vi "Periodic Tasks.vi"(8 "error in":errorcluster) -> ()   [LabVIEW 2019]
doc: "This VI runs in parallel to other tasks. It can contain as many user-defined periodic loops as you need. These can carry out PID or other sorts of timed response."
uses:
  <vilib>/Rock Robotics/WPI/DriverStation/WPI_DriverStationRobotMode2.ctl
  <vilib>/Rock Robotics/WPI/Utilities/WPI_GetSetVariantRefNum.vi
  Robot Global Data.vi
  <vilib>/Rock Robotics/Network Tables/NT Write Numeric Array.vi
  <vilib>/Rock Robotics/WPI/RobotDrive/WPI_RobotDriveArcadeDrive_Standard(NoSaturation).vi
  <vilib>/Rock Robotics/Network Tables/NT Write String.vi
  <vilib>/Rock Robotics/Network Tables/NT Write Number.vi
panel:
  in  "Yellow":cluster{"R":dbl, "G":dbl, "B":dbl}
  in  "Blue":cluster{"R":dbl, "G":dbl, "B":dbl}
  in  "Green":cluster{"R":dbl, "G":dbl, "B":dbl}
  in  "Red":cluster{"R":dbl, "G":dbl, "B":dbl}
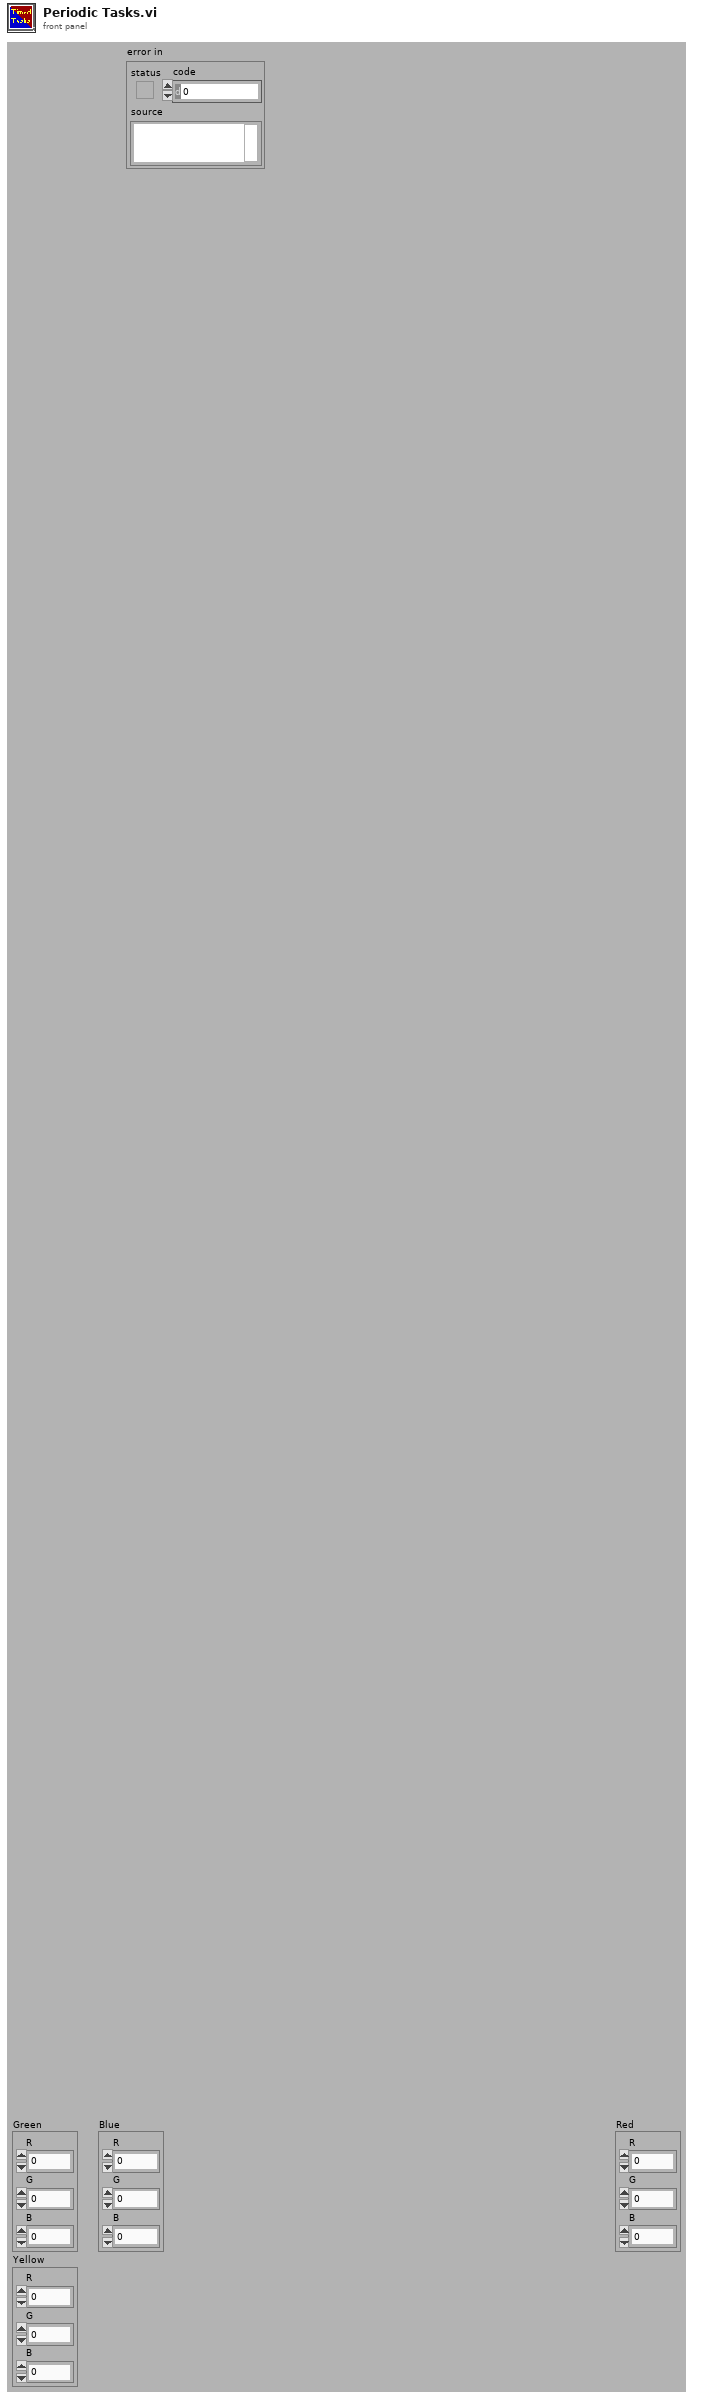
[diagram p1: front panel]
types:
  T1 = typedef "WPI_RobotDriveDevRef.ctl" = cluster{"DevStatus":errorcluster, "Motors[]":T2[], "Square Inputs":bool, "Max Output":dbl}
  T2 = typedef "WPI_MotorControlDeviceRef.ctl" = cluster{"DeviceStatus":errorcluster, "Type":T3, "PWM":cluster{"PWM Channel":T4, "DeadBand":T5}, "CAN":cluster{"Device Number":u8, "SetOutput VI Ref":variant, "GetOutput VI Ref":variant, "Enable VI Ref":variant, "Disable VI Ref":variant, "Data":variant}, "Invert":bool, "DIO PWM":cluster{"PWM \"Enable\" Channel":T4, "DIOChannel":T6, "PWM Rate":dbl}}
  T3 = typedef "WPI_MotorControlType.ctl" = enum16{"PWM", "CAN", "DIO PWM"}
  T4 = typedef "FPGA_DIOPWMChannel.ctl" = enum8{"PWM 0", "PWM 1", "PWM 2", "PWM 3", "PWM 4", "PWM 5", "PWM 6", "PWM 7", "PWM 8", "PWM 9", "PWM MXP 0", "PWM MXP 1", "PWM MXP 2", "PWM MXP 3", "PWM MXP 4", "PWM MXP 5", "PWM MXP 6", "PWM MXP 7", "PWM MXP 8", "PWM MXP 9", "Invalid"}
  T5 = typedef "WPI_PWMDeadband.ctl" = cluster{"Name":string, "maxPositivePwm":i32, "minPositivePwm":i32, "centerPwm":i32, "maxNegativePwm":i32, "minNegativePwm":i32, "angularRange":u16}
  T6 = typedef "FPGA_DIOChannel.ctl" = enum8{"DIO 0", "DIO 1", "DIO 2", "DIO 3", "DIO 4", "DIO 5", "DIO 6", "DIO 7", "DIO 8", "DIO 9", "DIO MXP 0", "DIO MXP 1", "DIO MXP 2", "DIO MXP 3", "DIO MXP 4", "DIO MXP 5", "DIO MXP 6", "DIO MXP 7", "DIO MXP 8", "DIO MXP 9", "DIO MXP 10", "DIO MXP 11", "DIO MXP 12", "DIO MXP 13", "DIO MXP 14", "DIO MXP 15", "SPI Port CS1", "SPI Port CS2", "SPI Port CS3", "SPI Port MISO", "SPI Port MOSI", "Invalid"}
  T7 = typedef "WPI_JoystickDevRef.ctl" = cluster{"Device":T8}
  T8 = typedef "WPI_JoystickDeviceEnum.ctl" = enum16{"USB 0", "USB 1", "USB 2", "USB 3", "USB 4", "USB 5"}
  T9 = cluster{"JoystickDevRef":T7, "RobotDriveDevRef":T1}
  T10 = typedef "Color Sensor V3 DevRef.ctl" = cluster{"I2CDevRef":T11}
  T11 = typedef "WPI_I2CDevRef.ctl" = cluster{"DevStatus":errorcluster, "Device Address":u8, "Handle":i32, "I2C Bus":T12}
  T12 = typedef "i2c_bus.ctl" = enum16{"I2C On-Board", "I2C MXP", "Invalid"}
  T13 = typedef "WPI_DriverStationRobotMode2.ctl" = enum16{"Autonomous Disabled", "Autonomous Enabled", "Teleop Disabled", "Teleop Enabled", "Disconnected", "Finish", "Test Disabled", "Test Enabled", "Emergency Stopped"}
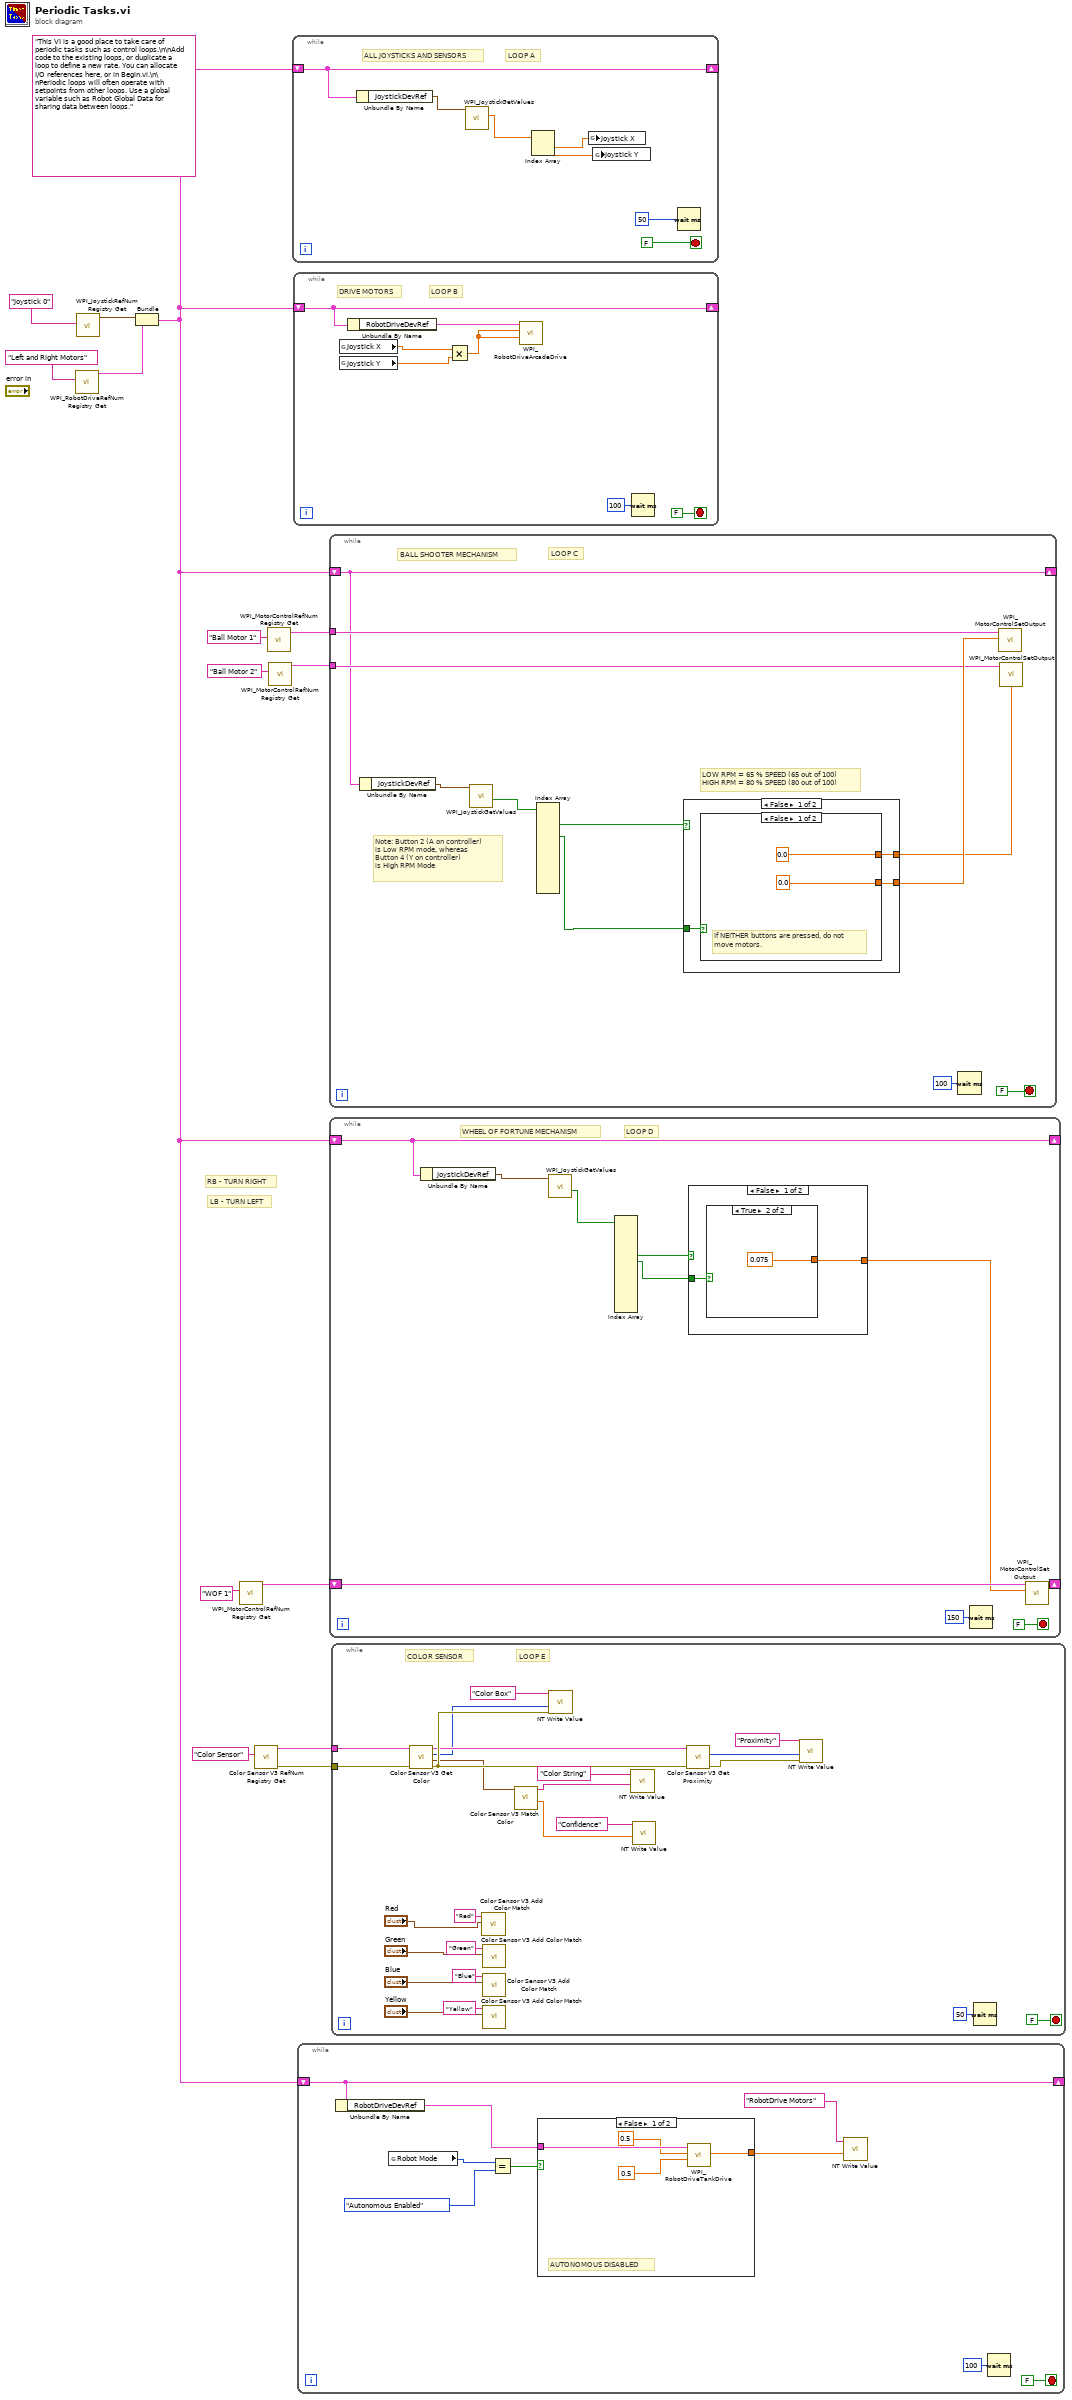
[diagram p0: block diagram]
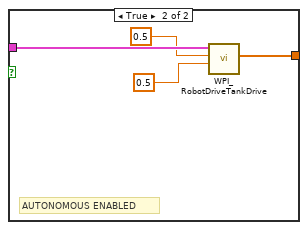
[diagram p2: hidden frame]
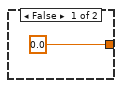
[diagram p3: hidden frame]
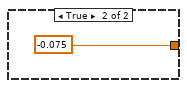
[diagram p4: hidden frame]
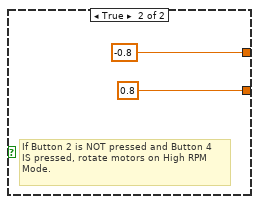
[diagram p5: hidden frame]
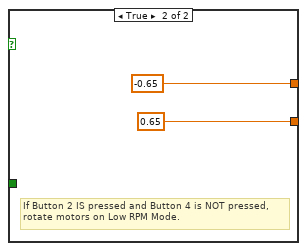
[diagram p6: hidden frame]
diagram:
  (unwired) "This VI is a good place to take care of periodic tasks such as control loops.\n\nAdd code to the existing loops, or duplicate a loop to define a new rate. You can allocate I/O references here, or in Begin.vi.\n\nPeriodic loops will often operate with setpoints from other loops. Use a global variable such as Robot Global Data for sharing data between loops."
  # "LB - TURN LEFT"
  # "RB - TURN RIGHT"
  n1 = call <vilib>:"WPI_RobotDriveRefNum Registry Get.vi"("refnum name"="Left and Right Motors") -> ("RobotDriveDevRef"=w11:T1)  [unwired: 1 in, 9 out]
  n2 = call <vilib>:"WPI_JoystickRefNum Registry Get.vi"("refnum name"="Joystick 0") -> ("JoystickDevRef"=w12:T7)  [unwired: 1 in, 9 out]
  n3 = Bundle("JoystickDevRef"=w12, "RobotDriveDevRef"=w11) -> (w1:T9)  [unwired: 1 out]
  n4 = call <vilib>:"WPI_MotorControlRefNum Registry Get.vi"("refnum name"="WOF 1") -> ("MotorControlDevRef"=w5:T2)  [unwired: 9 in, 1 out]
  n5 = call <vilib>:"Color Sensor V3 RefNum Registry Get.vi"("refnum name"="Color Sensor") -> ("error out"=w2:errorcluster, "ColorSensorDevRef"=w4:T10)  [unwired: 9 in]
  n6 = call <vilib>:"WPI_MotorControlRefNum Registry Get.vi"("refnum name"="Ball Motor 1") -> ("MotorControlDevRef"=w8:T2)  [unwired: 9 in, 1 out]
  n7 = call <vilib>:"WPI_MotorControlRefNum Registry Get.vi"("refnum name"="Ball Motor 2") -> ("MotorControlDevRef"=w7:T2)  [unwired: 9 in, 1 out]
  n8 = while {
    shift-right: [w20] -> _
    shift-left: w1 -> [w20]
    stop <- FALSE stop-if-true
    # "LOOP A"
    # "ALL JOYSTICKS AND SENSORS"
    n9 = Unbundle By Name(w20) -> ("JoystickDevRef"=w19:T7)
    n10 = call <vilib>:"WPI_JoystickGetValues.vi"("JoystickDevRef"=w19) -> ("Axes"=w18:dbl[])  [unwired: 6 in, 4 out]
    n11 = Index Array(array=w18) -> (element #1=w16:dbl, element #2=w17:dbl)  [unwired: 2 in]
    n12 = global write "Robot Global Data.vi" "Joystick X"(w16) -> ()
    n13 = global write "Robot Global Data.vi" "Joystick Y"(w17) -> ()
    n14 = Wait (ms)(milliseconds to wait=u32 50) -> ()  [unwired: 1 out]
  }
  n15 = while {
    shift-right: [w26] -> _
    shift-left: w1 -> [w26]
    stop <- FALSE stop-if-true
    # "LOOP B"
    # "DRIVE MOTORS"
    n16 = global read "Robot Global Data.vi" "Joystick X"() -> (w22:dbl)
    n17 = global read "Robot Global Data.vi" "Joystick Y"() -> (w23:dbl)
    n18 = Unbundle By Name(w26) -> ("RobotDriveDevRef"=w25:T1)
    n19 = Multiply(x=w22, y=w23) -> (x*y=w24:dbl)
    n20 = call-poly <vilib>:"WPI_RobotDriveArcadeDrive.vi"("Y axis value"=w24, "X axis value"=w24, "RobotDriveDevRef"=w25) -> ()  [unwired: 6 in, 3 out]
    n21 = Wait (ms)(milliseconds to wait=u32 100) -> ()  [unwired: 1 out]
  }
  n22 = while {
    shift-right: [w37] -> _
    shift-left: w1 -> [w37]
    stop <- FALSE stop-if-true
    n23 = Unbundle By Name(w37) -> ("RobotDriveDevRef"=w33:T1)
    n24 = global read "Robot Global Data.vi" "Robot Mode"() -> (w36:T13)
    n25 = Equal?(x=w36, y=WPI_DriverStationRobotMode2."Autonomous Enabled") -> (x = y?=w35:bool)
    n26 = case shown="False" w35 {
      tunnel: w33 -> [w40 w44]
      tunnel: [w41 w45] -> w29
      frame False {
        # "AUTONOMOUS DISABLED"
        n27 = call <vilib>:"WPI_RobotDriveTankDrive.vi"("Right axis value"=0.5, "Left axis value"=0.5, "RobotDriveDevRef"=w40) -> ("Motor Values"=w41:dbl[])  [unwired: 6 in, 2 out]
      }
      frame True {
        # "AUTONOMOUS ENABLED"
        n28 = call <vilib>:"WPI_RobotDriveTankDrive.vi"("Right axis value"=0.5, "Left axis value"=0.5, "RobotDriveDevRef"=w44) -> ("Motor Values"=w45:dbl[])  [unwired: 6 in, 2 out]
      }
    }
    n29 = call-poly <vilib>:"NT Write Value.vi"("Numeric Array"=w29, "Name"="RobotDrive Motors") -> ()  [unwired: 9 in, 1 out]
    n30 = Wait (ms)(milliseconds to wait=u32 100) -> ()  [unwired: 1 out]
  }
  n31 = while {
    shift-right: [w50] -> _
    shift-left: w1 -> [w50]
    tunnel: w8 -> [w54]
    tunnel: w7 -> [w51]
    stop <- FALSE stop-if-true
    # "LOW RPM = 65 % SPEED (65 out of 100)\nHIGH RPM = 80 % SPEED (80 out of 100)"
    # "LOOP C"
    # "Note: Button 2 (A on controller) \nis Low RPM mode, whereas \nButton 4 (Y on controller)\nis High RPM Mode"
    # "BALL SHOOTER MECHANISM"
    n32 = Unbundle By Name(w50) -> ("JoystickDevRef"=w49:T7)
    n33 = call <vilib>:"WPI_JoystickGetValues.vi"("JoystickDevRef"=w49) -> ("Buttons"=w48:bool[])  [unwired: 6 in, 4 out]
    n34 = Index Array(array=w48) -> (element #2=w46:bool, element #4=w47:bool)  [unwired: 13 in, 11 out]
    n35 = case shown="False" w46 {
      tunnel: [w59 0.65 ("Output")] -> w53
      tunnel: [w58 -0.65 ("Output")] -> w52
      tunnel: w47 -> [w57 _]
      frame False {
        n36 = case shown="False" w57 {
          tunnel: [0.0 ("Output") 0.8 ("Output")] -> w59
          tunnel: [0.0 ("Output") -0.8 ("Output")] -> w58
          frame False {
            # "If NEITHER buttons are pressed, do not\nmove motors."
          }
          frame True {
            # "If Button 2 is NOT pressed and Button 4\nIS pressed, rotate motors on High RPM\nMode."
          }
        }
      }
      frame True {
        # "If Button 2 IS pressed and Button 4 is NOT pressed,\nrotate motors on Low RPM Mode."
      }
    }
    n37 = Wait (ms)(milliseconds to wait=u32 100) -> ()  [unwired: 1 out]
    n38 = call <vilib>:"WPI_MotorControlSetOutput.vi"("Output"=w53, "MotorControlDevRef"=w54) -> ()  [unwired: 7 in, 3 out]
    n39 = call <vilib>:"WPI_MotorControlSetOutput.vi"("Output"=w52, "MotorControlDevRef"=w51) -> ()  [unwired: 7 in, 3 out]
  }
  n40 = while {
    shift-right: [w74] -> _
    shift-left: w1 -> [w74]
    shift-right: [w70] -> _
    shift-left: w5 -> [w71]
    stop <- FALSE stop-if-true
    # "LOOP D"
    # "WHEEL OF FORTUNE MECHANISM"
    n41 = Unbundle By Name(w74) -> ("JoystickDevRef"=w73:T7)
    n42 = call <vilib>:"WPI_JoystickGetValues.vi"("JoystickDevRef"=w73) -> ("Buttons"=w72:bool[])  [unwired: 6 in, 4 out]
    n43 = Index Array(array=w72) -> (element #5=w68:bool, element #6=w67:bool)  [unwired: 14 in, 12 out]
    n44 = case shown="False" w68 {
      tunnel: [w76 -0.075 ("Output")] -> w69
      tunnel: w67 -> [w77 _]
      frame False {
        n45 = case shown="True" w77 {
          tunnel: [0.0 ("Output") 0.075 ("Output")] -> w76
          frame False {
          }
          frame True {
          }
        }
      }
      frame True {
      }
    }
    n46 = Wait (ms)(milliseconds to wait=u32 150) -> ()  [unwired: 1 out]
    n47 = call <vilib>:"WPI_MotorControlSetOutput.vi"("Output"=w69, "MotorControlDevRef"=w71) -> ("MotorControlDevRef"=w70:T2)  [unwired: 7 in, 2 out]
  }
  n48 = while {
    tunnel: w4 -> [w103]
    tunnel: w2 -> [w102]
    stop <- FALSE stop-if-true
    # "LOOP E"
    # "COLOR SENSOR"
    n49 = call <vilib>:"Color Sensor V3 Get Color.vi"("error in (no error)"=w102, "ColorSensorDevRef"=w103) -> ("error out"=w101:errorcluster, "Normalized Color"=w95:cluster{"R":dbl, "G":dbl, "B":dbl}, "Color"=w98:u32, "ColorSensorDevRef out"=w99:T10)  [unwired: 6 in]
    n50 = call <vilib>:"Color Sensor V3 Add Color Match.vi"("Color"="Red", "Name"="Red") -> ()  [unwired: 10 in]
    n51 = call <vilib>:"Color Sensor V3 Add Color Match.vi"("Color"="Green", "Name"="Green") -> ()  [unwired: 10 in]
    n52 = call <vilib>:"Color Sensor V3 Add Color Match.vi"("Color"="Blue", "Name"="Blue") -> ()  [unwired: 10 in]
    n53 = call <vilib>:"Color Sensor V3 Add Color Match.vi"("Color"="Yellow", "Name"="Yellow") -> ()  [unwired: 10 in]
    n54 = call <vilib>:"Color Sensor V3 Match Color.vi"("Measured Color"=w95) -> ("Confidence"=w94:dbl, "Matched Color Name"=w93:string)  [unwired: 8 in, 1 out]
    n55 = call-poly <vilib>:"NT Write Value.vi"("error in"=w101, "Numeric"=w98, "Name"="Color Box") -> ()  [unwired: 8 in, 1 out]
    n56 = call-poly <vilib>:"NT Write Value.vi"("String"=w93, "Name"="Color String") -> ()  [unwired: 9 in, 1 out]
    n57 = call-poly <vilib>:"NT Write Value.vi"("Numeric"=w94, "Name"="Confidence") -> ()  [unwired: 9 in, 1 out]
    n58 = call <vilib>:"Color Sensor V3 Get Proximity.vi"("error in (no error)"=w101, "ColorSensorDevRef"=w99) -> ("error out"=w96:errorcluster, "Proximity"=w97:u16)  [unwired: 7 in, 1 out]
    n59 = call-poly <vilib>:"NT Write Value.vi"("error in"=w96, "Numeric"=w97, "Name"="Proximity") -> ()  [unwired: 8 in, 1 out]
    n60 = Wait (ms)(milliseconds to wait=u32 50) -> ()  [unwired: 1 out]
  }
